vi "test_nameCluster.vi"() -> ()   [LabVIEW 2013]
uses:
  <vilib>/Utility/GetType.llb/TD_Create Cluster.vi
  source/Variant/OpenVariant.lvlib
panel:
  out "Cluster":variant
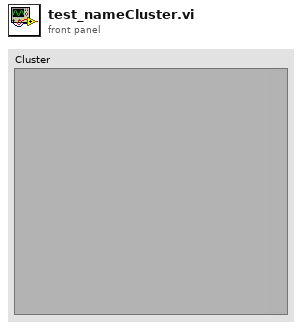
[diagram p1: front panel]
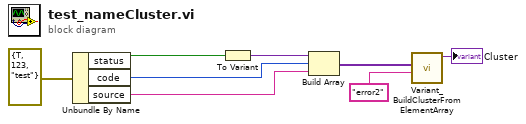
[diagram p0: block diagram]
diagram:
  n1 = Unbundle By Name(errorcluster {"status"=TRUE, "code"=123, "source"="test"} ("error constant")) -> ("status"=w6:bool, "code"=w5:i32, "source"=w4:string)
  n2 = To Variant(anything=w6) -> (Variant=w8:variant)
  n3 = Build Array(w8, w5, w4) -> (w2:variant[])
  n4 = call "Variant_BuildClusterFromElementArray.vi"("name"="error2", "Elements"=w2) -> ("Cluster"=→"Cluster":variant)  [unwired: 9 in]
